vi "Encode Close Payload.vi"(8 "error in (no error)":errorcluster, 11 "Code":u32) -> (0 "error out":errorcluster, 3 "Packet":string)   [LabVIEW 2023, in "WebSocket.lvclass"]
uses:
  WebSocket.lvclass
  private/Fixed Header.ctl
  private/OpCode.ctl
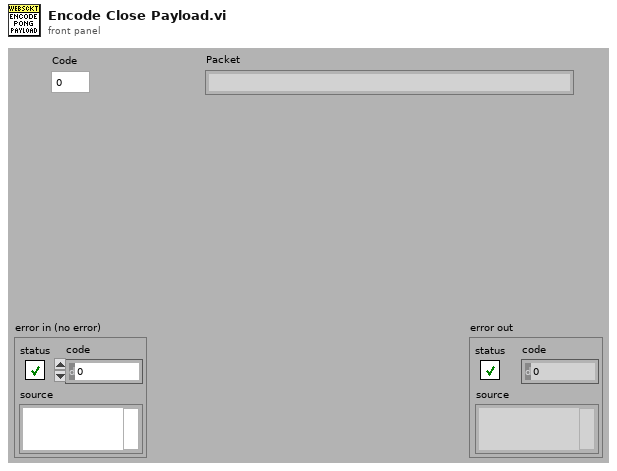
[diagram p1: front panel]
types:
  T1 = typedef "WebSocket.lvclass/Fixed Header.ctl" = cluster{"FIN":bool, "RSVD1":bool, "RSVD2":bool, "RSVD3":bool, "OpCode":T2, "MASK":bool, "Len":u8}
  T2 = typedef "WebSocket.lvclass/OpCode.ctl" = enum16{"Cont.", "Text", "Binary", "NonCtl3", "NonCtl4", "NonCtl5", "NonCtl6", "NonCtl7", "Close", "Ping", "Pong", "Rsvd11", "Rsvd12", "Rsvd13", "Rsvd14", "Rsvd15"}
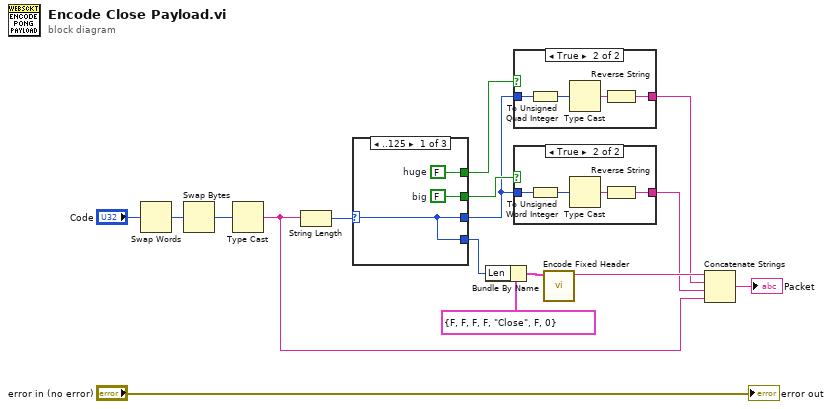
[diagram p0: block diagram]
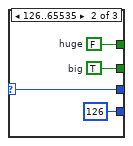
[diagram p4: hidden frame]
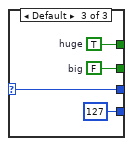
[diagram p5: hidden frame]
diagram:
  n1 = Swap Words(1:"Code") -> (0:w3:u32)
  n2 = Swap Bytes(anything=w3) -> (byte swapped=w2:u32)
  n3 = Type Cast(x=w2) -> (*(type *) &x=w1:string)  [unwired: 1 in]
  n4 = String Length(string=w1) -> (length=w15:i32)
  n5 = case shown="..125" w15 {
    selector: w15 -> [w17 w23 w27]
    tunnel: [w17 w23 w27] -> w10
    tunnel: [w19 w22 w26] -> w11
    tunnel: [w18 w21 w25] -> w12
    tunnel: [w17 126 ("Len") 127 ("Len")] -> w13
    frame ..125 {
      w19 = FALSE  # big
      w18 = FALSE  # huge
    }
    frame 126..65535 {
      w22 = TRUE  # big
      w21 = FALSE  # huge
    }
    frame Default {
      w26 = FALSE  # big
      w25 = TRUE  # huge
    }
  }
  n6 = Bundle By Name(cluster=T1 {"FIN"=FALSE, "RSVD1"=FALSE, "RSVD2"=FALSE, "RSVD3"=FALSE, "OpCode"=enum."Close", "MASK"=FALSE, "Len"=0} ("Fixed Header"), "Len"=w13) -> (w14:T1)
  n7 = case shown="True" w12 {
    tunnel: w10 -> [_ w31]
    tunnel: [_ w28] -> w8
    frame False {
    }
    frame True {
      n8 = To Unsigned Quad Integer(1:w31) -> (0:w30:u64)
      n9 = Type Cast(x=w30) -> (*(type *) &x=w29:string)  [unwired: 1 in]
      n10 = Reverse String(1:w29) -> (0:w28:string)
    }
  }
  n11 = case shown="True" w11 {
    tunnel: w10 -> [_ w35]
    tunnel: [_ w32] -> w7
    frame False {
    }
    frame True {
      n12 = To Unsigned Word Integer(number=w35) -> (unsigned 16bit integer=w34:u16)
      n13 = Type Cast(x=w34) -> (*(type *) &x=w33:string)  [unwired: 1 in]
      n14 = Reverse String(1:w33) -> (0:w32:string)
    }
  }
  n15 = call "Encode Fixed Header.vi"("Fixed Header"=w14) -> ("String"=w9:string)  [unwired: 9 in, 1 out]
  n16 = Concatenate Strings(w9, w8, w7, w1) -> (→"Packet":string)
  "error out" <- "error in (no error)"
